vi "Controller Process.vi"(8 "error in (no error)":errorcluster, 11 "View Model":T1) -> (0 "error out":errorcluster)   [LabVIEW 2017]
doc: "This is the SW component that allows the user to interact with the controls and provides appropriate feedback as requested through the displa console."
uses:
  View Model/Controls/View Model.ctl
  View Model/Controls/Shared Model.ctl
  Error Handler/Controls/Error Model.ctl
  Error Handler/Controls/Error Message.ctl
  Error Handler/Controls/Error Level.ctl
  Configuration/Controls/Database Model.ctl
  Configuration/Controls/Database Message.ctl
  Configuration/Controls/Database Command.ctl
  Configuration/Controls/Database Overhead.ctl
  Configuration/Controls/Database Status.ctl
  Configuration/Controls/Database Record.ctl
  Configuration/Controls/Database - Rule Record.ctl
  Controls/CNTRLR - Wash Step.ctl
  Controls/CNTRLR - Position.ctl
  Controls/CNTRLR - Model.ctl
  Controls/CNTRLR - Message.ctl
  Controls/CNTRLR - Command.ctl
  Controls/CNTRLR - Overhead.ctl
  Controls/CNTRLR - State.ctl
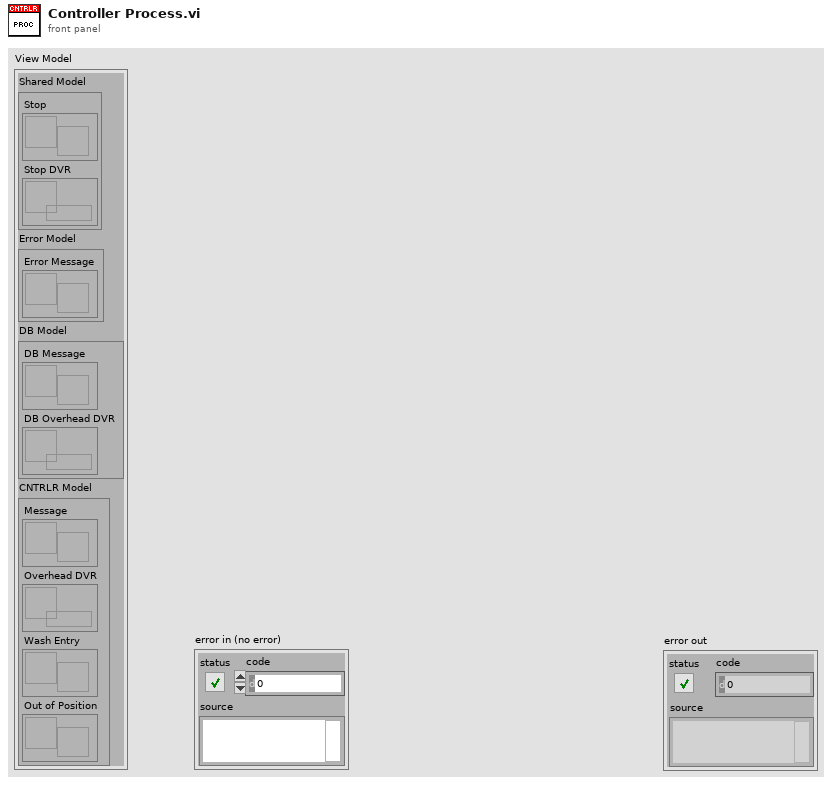
[diagram p1: front panel]
types:
  T1 = typedef "View Model.ctl" = cluster{"Shared Model":T2, "Error Model":T3, "DB Model":T4, "CNTRLR Model":T5}
  T2 = typedef "Shared Model.ctl" = cluster{"Stop":refnum<user-event>, "Stop DVR":refnum<data-value>}
  T3 = typedef "Error Model.ctl" = cluster{"Error Message":refnum<user-event>}
  T4 = typedef "Database Model.ctl" = cluster{"DB Message":refnum<user-event>, "DB Overhead DVR":refnum<data-value>}
  T5 = typedef "CNTRLR - Model.ctl" = cluster{"Message":refnum<user-event>, "Overhead DVR":refnum<data-value>, "Wash Entry":refnum<user-event>, "Out of Position":refnum<user-event>}
  T6 = typedef "CNTRLR - State.ctl" = enum16{"Initial", "Wait for Start", "Start State", "Wait for Vehicle Position", "Wash Step Execution", "Wash Step/Cycle Complete", "Wash Exit", "Wash Abort/Terminate"}
  T7 = typedef "CNTRLR - Command.ctl" = enum16{"Idle", "Start Car Wash", "Error", "Stop"}
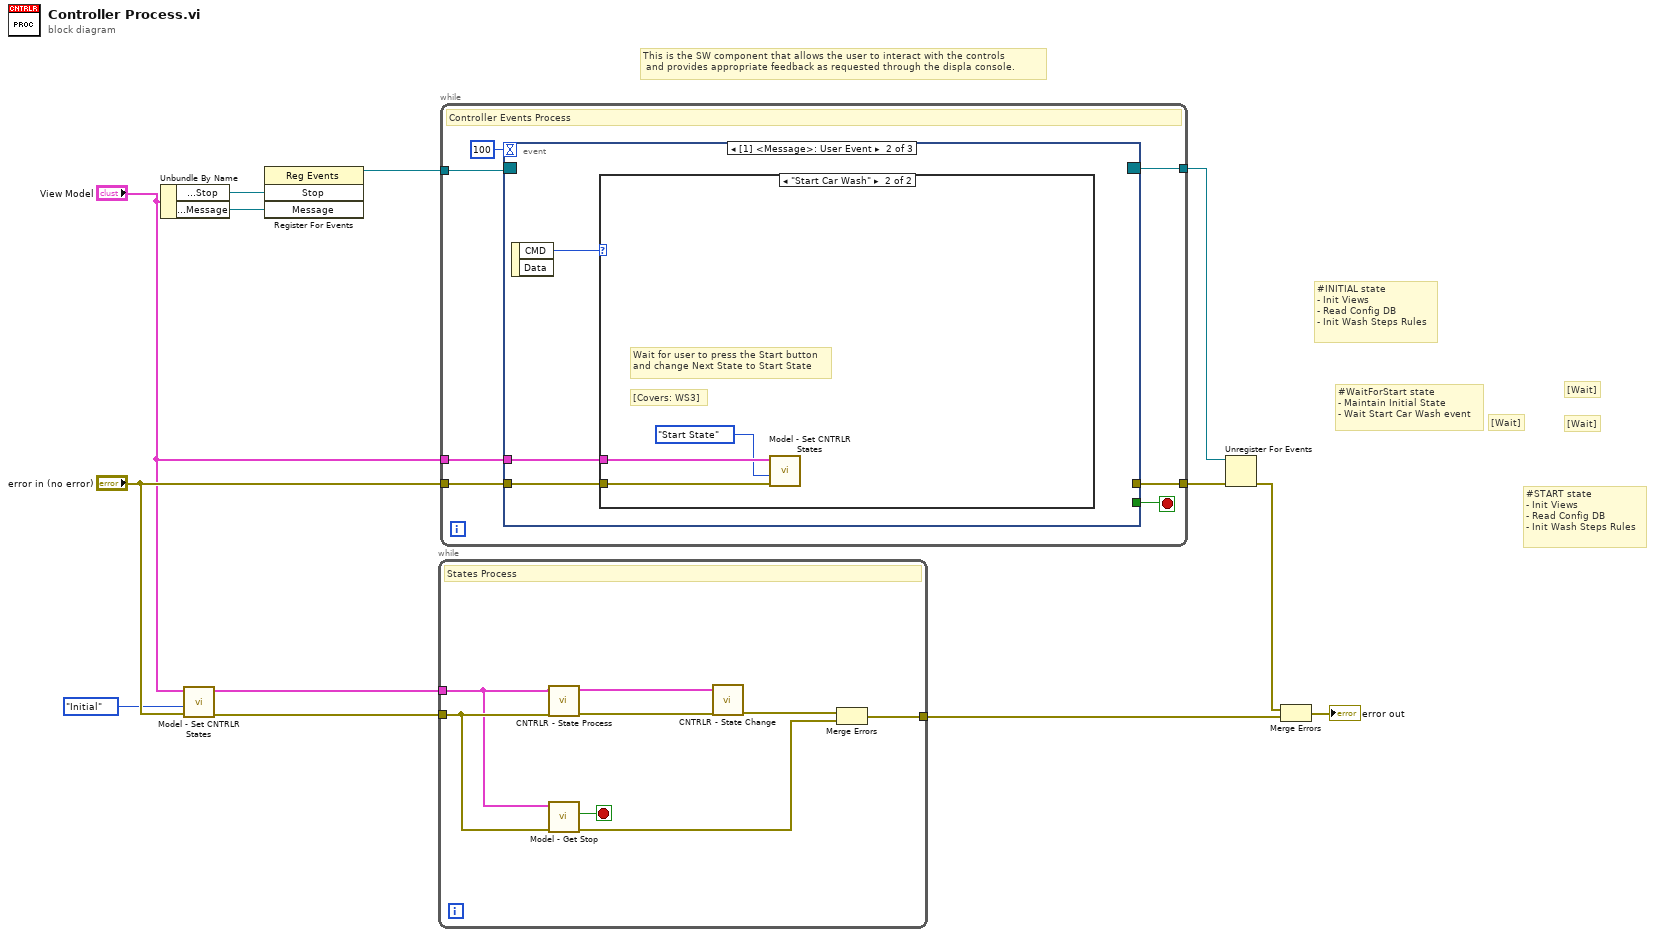
[diagram p0: block diagram]
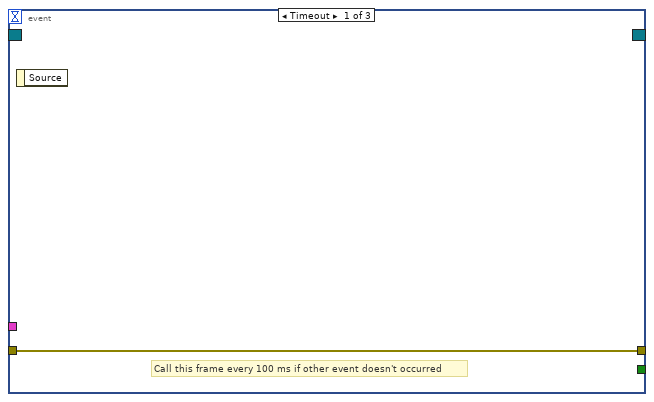
[diagram p2: hidden frame]
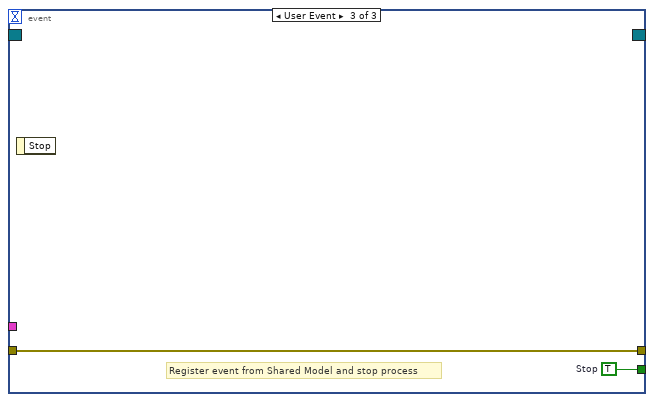
[diagram p4: hidden frame]
diagram:
  # "#START state\n- Init Views\n- Read Config DB\n- Init Wash Steps Rules"
  # "[Wait]"
  # "[Wait]"
  # "[Wait]"
  # "#WaitForStart state\n- Maintain Initial State\n- Wait Start Car Wash event"
  # "#INITIAL state\n- Init Views\n- Read Config DB\n- Init Wash Steps Rules"
  # "This is the SW component that allows the user to interact with the controls\n and provides appropriate feedback as requested through the displa console."
  n1 = Unbundle By Name("View Model") -> ("Shared Model.Stop"=w13:refnum<user-event>, "CNTRLR Model.Message"=w2:refnum<user-event>)
  n2 = call "Model - Set CNTRLR States.vi"("error in (no error)"="error in (no error)", "Next State"=CNTRLR_-_State."Initial", "View Model"="View Model") -> ("error out"=w3:errorcluster, "View Model"=w4:T1)  [unwired: 7 in]
  n3 = register-events(w13, w2) -> (reference out=w12:refnum<event-registration>)  [unwired: 2 in, 1 out]
  n4 = while {
    tunnel: w3 -> [w20]
    tunnel: [w14] -> w9
    tunnel: w4 -> [w19]
    stop <- w21 stop-if-true
    # "States Process"
    n5 = call "CNTRLR - State Process.vi"("error in (no error)"=w20, "View Model"=w19) -> ("error out"=w18:errorcluster, "View Model"=w17:T1)  [unwired: 8 in]
    n6 = call "Model - Get Stop.vi"("error in (no error)"=w20, "View Model"=w19) -> ("error out"=w15:errorcluster, "Stop"=w21:bool)  [unwired: 7 in, 1 out]
    n7 = call "CNTRLR - State Change.vi"("error in (no error)"=w18, "View Model"=w17) -> ("error out"=w16:errorcluster)  [unwired: 8 in, 1 out]
    n8 = Merge Errors(w16, w15) -> (w14:errorcluster)
  }
  n9 = while {
    tunnel: w12 -> [w28]
    tunnel: "error in (no error)" -> [w27]
    tunnel: [w26] -> w10
    tunnel: [w23] -> w11
    tunnel: "View Model" -> [w22]
    stop <- w24 stop-if-true
    # "Controller Events Process"
    n10 = event shown="[1] <Message>: User Event" {
      selector: w28 -> [_ _ _]
      dyn-events: [_ _ _] -> w23
      timeout: 100 -> [_ _ _]
      tunnel: w27 -> [w29 w31 w36]
      tunnel: [w29 _ w36] -> w26
      tunnel: [_ _ w37] -> w24
      tunnel: w22 -> [_ w30 _]
      event Timeout {
        # "Call this frame every 100 ms if other event doesn't occurred"
        n11 = event-data() -> ()  [unwired: 1 in, 1 out]
      }
      event User Event {
        n12 = event-data() -> ("CMD"=w32:T7)  [unwired: 1 in, 1 out]
        n13 = case shown="\"Start Car Wash\"" w32 {
          tunnel: w31 -> [_ w35]
          tunnel: w30 -> [_ w34]
          frame "Idle", Default {
          }
          frame "Start Car Wash" {
            # "[Covers: WS3]"
            # "Wait for user to press the Start button\nand change Next State to Start State"
            n14 = call "Model - Set CNTRLR States.vi"("error in (no error)"=w35, "Next State"=CNTRLR_-_State."Start State", "View Model"=w34) -> ()  [unwired: 7 in, 2 out]
          }
        }
      }
      event User Event {
        w37 = TRUE  # Stop
        # "Register event from Shared Model and stop process"
        n15 = event-data() -> ()  [unwired: 1 in, 1 out]
      }
    }
  }
  n16 = Unregister For Events(event registration refnum=w11, error in=w10) -> (error out=w8:errorcluster)
  n17 = Merge Errors(w8, w9) -> (→"error out":errorcluster)
